vi "MBcrc.vi"(10 "Data in:":u8[](array[numeric]) format="%.0x") -> (2 "Data out:":string, 3 "CRC":u16 format="%.0x")   [LabVIEW 2010]
doc: "VI calculates CRC for Modbus protocol"
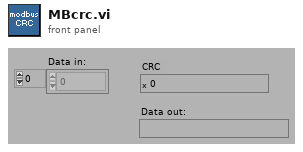
[diagram p1: front panel]
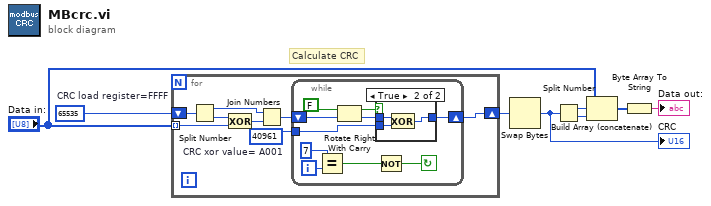
[diagram p0: block diagram]
diagram:
  w5 = u16 65535  # CRC load register=FFFF
  # "Calculate CRC"
  n1 = for {
    tunnel: "Data in:" -> [w15] mode=indexing
    shift-right: [w14] -> w4
    shift-left: w5 -> [w16]
    w9 = u16 40961  # CRC xor value= A001
    n2 = Split Number(x=w16) -> (hi(x)=w10:u8, lo(x)=w12:u8)
    n3 = Exclusive Or(1:w15, 2:w12) -> (0:w11:u8)
    n4 = Join Numbers(hi=w10, lo=w11) -> ((hi.lo)=w13:u16)
    n5 = while {
      shift-left: w13 -> [w22]
      shift-right: [w23] -> w14
      tunnel: w9 -> [w25]
      i -> [w20]
      stop <- w24 continue-if-true
      n6 = Equal?(x=7, y=w20) -> (x = y?=w18:bool)
      n7 = Rotate Right With Carry(2:w22, 3:FALSE) -> (0:w17:u16, 1:w19:bool)
      n8 = case shown="True" w19 {
        tunnel: w17 -> [w27 w30]
        tunnel: w25 -> [_ w29]
        tunnel: [w27 w28] -> w23
        frame False {
        }
        frame True {
          n9 = Exclusive Or(1:w29, 2:w30) -> (0:w28:u16)
        }
      }
      n10 = Not(x=w18) -> (.not. x?=w24:bool)
    }
  }
  n11 = Swap Bytes(anything=w4) -> (byte swapped=w1:u16)
  "CRC" <- w1
  n12 = Split Number(x=w1) -> (hi(x)=w3:u8, lo(x)=w2:u8)
  n13 = Build Array (concatenate)("Data in:", w3, w2) -> (w8:u8[])
  n14 = Byte Array To String(unsigned byte array=w8) -> (string=→"Data out:":string)
